vi "Read Encoders.vi"(8 "error in":errorcluster, 11 "TeleOp Data Cluster in":T1) -> (0 "error out":errorcluster, 3 "TeleOp Data Cluster out":T1)   [LabVIEW 2018]
uses:
  TypeDefs/Teleop Data Cluster.ctl
  TypeDefs/typedef_enum_Refnums.ctl
  <vilib>/Rock Robotics/WPI/ThirdParty/Phoenix-LabVIEW/Motor Controller/Get/CTRE_Phoenix_MotorController_GetQuadratureData.vi
  <vilib>/Rock Robotics/WPI/ThirdParty/Phoenix-LabVIEW/Motor Controller/Get/CTRE_Phoenix_MotorController_GetLimitSwitchStates.vi
  <vilib>/Rock Robotics/WPI/ThirdParty/Phoenix-LabVIEW/Motor Controller/Get/CTRE_Phoenix_MotorController_GetVoltage.vi
  <vilib>/Rock Robotics/WPI/ThirdParty/Phoenix-LabVIEW/Motor Controller/Get/CTRE_Phoenix_MotorController_GetSelectedSensorData.vi
  <vilib>/Rock Robotics/Network Tables/NT Write Number.vi
  <vilib>/Rock Robotics/Network Tables/NT Write Boolean.vi
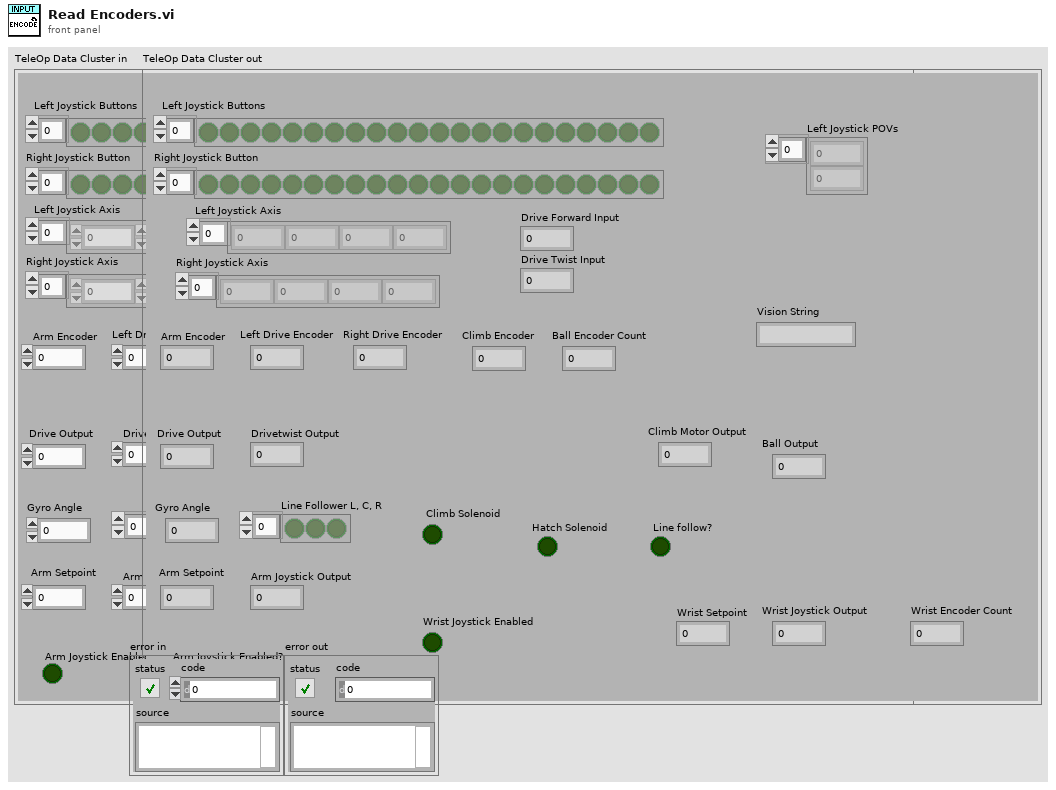
[diagram p1: front panel]
types:
  T1 = typedef "Teleop Data Cluster.ctl" = cluster{"Drive Forward Input ":dbl, "Drive Twist Input":dbl, "Drive Output":dbl, "Drivetwist Output":dbl, "Left Joystick Buttons":bool[], "Left Joystick Axis":dbl[], "Right Joystick Axis":dbl[], "Right Joystick Button":bool[], "Arm Encoder":dbl, "Left Drive Encoder":dbl, "Right Drive Encoder":dbl, "Gyro Angle ":dbl, "Arm Joystick Output  ":dbl, "Line Follower L, C, R ":bool[], "Line follow?":bool, " Climb Solenoid":bool, "Wrist Encoder Count":dbl, "Wrist Joystick Output":dbl, "Ball Encoder Count":dbl, "Ball Output":dbl, "Climb Encoder":dbl, "Climb Motor Output":dbl, " Hatch Solenoid":bool, "Arm Setpoint ":dbl, "Wrist Setpoint ":dbl, "Arm Joystick Enabled?":bool, "Wrist Joystick Enabled":bool, "Vision String":string, "Left Joystick POVs":i16[]}
  T2 = typedef "typedef_enum_Refnums.ctl" = enum16{"Ball_Encoder", "Ball_Motor", "Camera", "Linefollow_3", "Linefollow_2", "Linefollow_1", "Gyro", "Hatch_Solenoid", "Climb_Back_Solenoid", "Arm_Encoder", "Arm_Motor", "Lift_Encoder", "Drive", "Drive_Motor_R", "Drive_Motor_L", "Drive_Encoder_R", "Drive_Encoder_L", "Joy_R", "Joy_L", "Wrist_Motor", "Wrist_Encoder", "Climb Upper Limit", "Climb Lower Limit ", "Climb_Front_Motor"}
  T3 = typedef "WPI_MotorControlDeviceRef.ctl" = cluster{"DeviceStatus":errorcluster, "Type":T4, "PWM":cluster{"PWM Channel":T5, "DeadBand":T6}, "CAN":cluster{"Device Number":u8, "SetOutput VI Ref":variant, "GetOutput VI Ref":variant, "Enable VI Ref":variant, "Disable VI Ref":variant, "Data":variant}, "Invert":bool, "DIO PWM":cluster{"PWM \"Enable\" Channel":T5, "DIOChannel":T7, "PWM Rate":dbl}}
  T4 = typedef "WPI_MotorControlType.ctl" = enum16{"PWM", "CAN", "DIO PWM"}
  T5 = typedef "FPGA_DIOPWMChannel.ctl" = enum8{"PWM 0", "PWM 1", "PWM 2", "PWM 3", "PWM 4", "PWM 5", "PWM 6", "PWM 7", "PWM 8", "PWM 9", "PWM MXP 0", "PWM MXP 1", "PWM MXP 2", "PWM MXP 3", "PWM MXP 4", "PWM MXP 5", "PWM MXP 6", "PWM MXP 7", "PWM MXP 8", "PWM MXP 9", "Invalid"}
  T6 = typedef "WPI_PWMDeadband.ctl" = cluster{"Name":string, "maxPositivePwm":i32, "minPositivePwm":i32, "centerPwm":i32, "maxNegativePwm":i32, "minNegativePwm":i32, "angularRange":u16}
  T7 = typedef "FPGA_DIOChannel.ctl" = enum8{"DIO 0", "DIO 1", "DIO 2", "DIO 3", "DIO 4", "DIO 5", "DIO 6", "DIO 7", "DIO 8", "DIO 9", "DIO MXP 0", "DIO MXP 1", "DIO MXP 2", "DIO MXP 3", "DIO MXP 4", "DIO MXP 5", "DIO MXP 6", "DIO MXP 7", "DIO MXP 8", "DIO MXP 9", "DIO MXP 10", "DIO MXP 11", "DIO MXP 12", "DIO MXP 13", "DIO MXP 14", "DIO MXP 15", "SPI Port CS1", "SPI Port CS2", "SPI Port CS3", "SPI Port MISO", "SPI Port MOSI", "Invalid"}
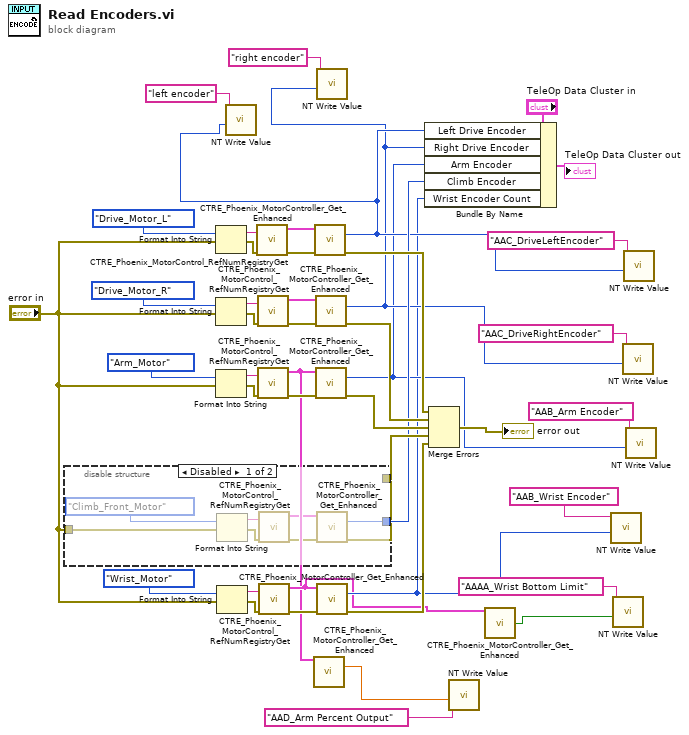
[diagram p0: block diagram]
diagram:
  n1 = disable-structure shown="Disabled" {
    disable-tunnel: "error in" -> [w47 _]
    disable-tunnel: [w46 _] -> w23
    disable-tunnel: [w45 _] -> w21
    frame Disabled {
      n2 = Format Into String(error in=w47, typedef_enum_Refnums."Climb_Front_Motor" ("RefNums")) -> (resulting string=w49:string, error out=w48:errorcluster)  [unwired: 2 in]
      n3 = call <vilib>:"CTRE_Phoenix_MotorControl_RefNumRegistryGet.vi"("error in (no error)"=w48, "refnum name"=w49) -> ("error out"=w51:errorcluster, "PhoenixMotorControlDevRef"=w50:T3)  [unwired: 8 in]
      n4 = call-poly <vilib>:"CTRE_Phoenix_MotorController_Get_Enhanced.vi"("PhoenixMotorControlDevRef"=w50, "error in"=w51) -> ("Quadrature Position"=w45:i32, "error out"=w46:errorcluster)  [unwired: 10 in, 2 out]
    }
    frame Enabled {
    }
  }
  n5 = Format Into String(error in="error in", typedef_enum_Refnums."Drive_Motor_L" ("RefNums")) -> (resulting string=w41:string, error out=w29:errorcluster)  [unwired: 2 in]
  n6 = Format Into String(error in="error in", typedef_enum_Refnums."Drive_Motor_R" ("RefNums")) -> (resulting string=w35:string, error out=w30:errorcluster)  [unwired: 2 in]
  n7 = Format Into String(error in="error in", typedef_enum_Refnums."Arm_Motor" ("RefNums")) -> (resulting string=w19:string, error out=w17:errorcluster)  [unwired: 2 in]
  n8 = Format Into String(error in="error in", typedef_enum_Refnums."Wrist_Motor" ("RefNums")) -> (resulting string=w27:string, error out=w25:errorcluster)  [unwired: 2 in]
  n9 = call <vilib>:"CTRE_Phoenix_MotorControl_RefNumRegistryGet.vi"("error in (no error)"=w29, "refnum name"=w41) -> ("error out"=w40:errorcluster, "PhoenixMotorControlDevRef"=w39:T3)  [unwired: 8 in]
  n10 = call <vilib>:"CTRE_Phoenix_MotorControl_RefNumRegistryGet.vi"("error in (no error)"=w30, "refnum name"=w35) -> ("error out"=w37:errorcluster, "PhoenixMotorControlDevRef"=w36:T3)  [unwired: 8 in]
  n11 = call <vilib>:"CTRE_Phoenix_MotorControl_RefNumRegistryGet.vi"("error in (no error)"=w17, "refnum name"=w19) -> ("error out"=w18:errorcluster, "PhoenixMotorControlDevRef"=w3:T3)  [unwired: 8 in]
  n12 = call <vilib>:"CTRE_Phoenix_MotorControl_RefNumRegistryGet.vi"("error in (no error)"=w25, "refnum name"=w27) -> ("error out"=w26:errorcluster, "PhoenixMotorControlDevRef"=w4:T3)  [unwired: 8 in]
  n13 = call-poly <vilib>:"CTRE_Phoenix_MotorController_Get_Enhanced.vi"("PhoenixMotorControlDevRef"=w3) -> ("Percent Output"=w2:dbl)  [unwired: 10 in, 4 out]
  n14 = call-poly <vilib>:"CTRE_Phoenix_MotorController_Get_Enhanced.vi"("PhoenixMotorControlDevRef"=w39, "error in"=w40) -> ("Quadrature Position"=w12:i32, "error out"=w34:errorcluster)  [unwired: 10 in, 2 out]
  n15 = call-poly <vilib>:"NT Write Value.vi"("Numeric"=w12, "Name"="left encoder") -> ()  [unwired: 9 in, 1 out]
  n16 = call-poly <vilib>:"CTRE_Phoenix_MotorController_Get_Enhanced.vi"("PhoenixMotorControlDevRef"=w36, "error in"=w37) -> ("Quadrature Position"=w11:i32, "error out"=w33:errorcluster)  [unwired: 10 in, 2 out]
  n17 = call-poly <vilib>:"CTRE_Phoenix_MotorController_Get_Enhanced.vi"("PhoenixMotorControlDevRef"=w3, "error in"=w18) -> ("Position (Raw Sensor Units)"=w10:i32, "error out"=w32:errorcluster)  [unwired: 10 in, 2 out]
  n18 = call-poly <vilib>:"NT Write Value.vi"("Numeric"=w11, "Name"="right encoder") -> ()  [unwired: 9 in, 1 out]
  n19 = call-poly <vilib>:"CTRE_Phoenix_MotorController_Get_Enhanced.vi"("PhoenixMotorControlDevRef"=w4, "error in"=w26) -> ("Quadrature Position"=w7:i32, "error out"=w22:errorcluster)  [unwired: 10 in, 2 out]
  n20 = Bundle By Name(cluster="TeleOp Data Cluster in", "Left Drive Encoder"=w12, "Right Drive Encoder"=w11, "Arm Encoder"=w10, "Climb Encoder"=w21, "Wrist Encoder Count"=w7) -> (→"TeleOp Data Cluster out":T1)
  n21 = Merge Errors(w34, w33, w32, w23, w22) -> (→"error out":errorcluster)
  n22 = call-poly <vilib>:"NT Write Value.vi"("Numeric"=w2, "Name"="AAD_Arm Percent Output") -> ()  [unwired: 9 in, 1 out]
  n23 = call-poly <vilib>:"CTRE_Phoenix_MotorController_Get_Enhanced.vi"("PhoenixMotorControlDevRef"=w4) -> ("Reverse Limit Closed?"=w5:bool)  [unwired: 11 in, 3 out]
  n24 = call-poly <vilib>:"NT Write Value.vi"("Numeric"=w7, "Name"="AAB_Wrist Encoder") -> ()  [unwired: 9 in, 1 out]
  n25 = call-poly <vilib>:"NT Write Value.vi"("Boolean"=w5, "Name"="AAAA_Wrist Bottom Limit") -> ()  [unwired: 9 in, 1 out]
  n26 = call-poly <vilib>:"NT Write Value.vi"("Numeric"=w11, "Name"="AAC_DriveRightEncoder") -> ()  [unwired: 9 in, 1 out]
  n27 = call-poly <vilib>:"NT Write Value.vi"("Numeric"=w12, "Name"="AAC_DriveLeftEncoder") -> ()  [unwired: 9 in, 1 out]
  n28 = call-poly <vilib>:"NT Write Value.vi"("Numeric"=w10, "Name"="AAB_Arm Encoder") -> ()  [unwired: 9 in, 1 out]
